vi "修改绑定信息.vi"(9 "修改信息":cluster{"职类":i32, "姓名":string}, 10 "用户名":string, 11 "数据库连接引用":T1) -> (0 "error out":errorcluster)   [LabVIEW 2013, in "数据库操作.lvclass"]
uses:
  <vilib>/addons/database/Connection.llb/Conn ObjectReference.ctl
  <vilib>/addons/database/Connection.llb/Conn Execute.vi
  <vilib>/addons/database/NI_Database_API.lvlib
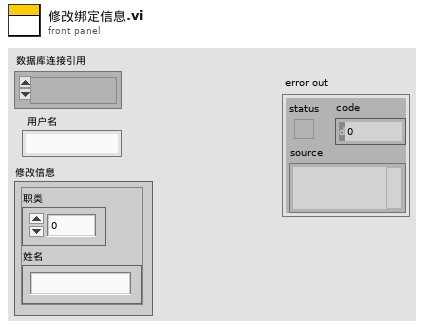
[diagram p1: front panel]
types:
  T1 = typedef "NI_Database_API.lvlib/Conn ObjectReference.ctl" = refnum<k1>
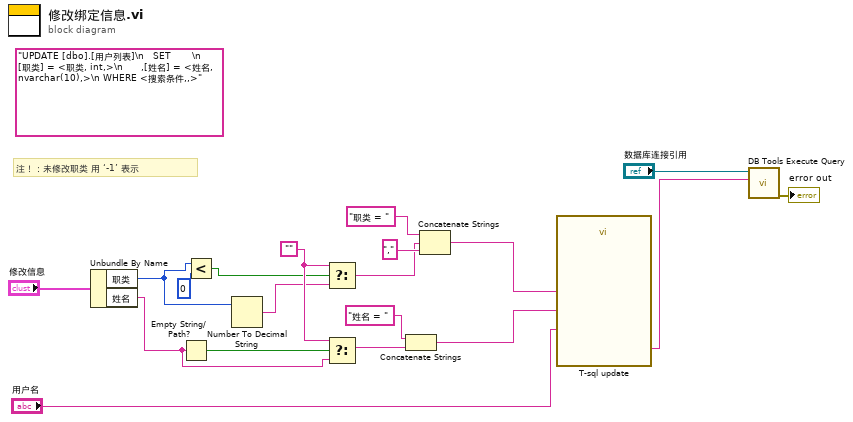
[diagram p0: block diagram]
diagram:
  w17 = ""
  (unwired) "UPDATE [dbo].[用户列表]\n   SET       \n      [职类] = <职类, int,>\n      ,[姓名] = <姓名, nvarchar(10),>\n WHERE <搜索条件,,>"
  # "注！：未修改职类 用 ‘-1’ 表示"
  n1 = Unbundle By Name("修改信息") -> ("职类"=w14:i32, "姓名"=w12:string)
  n2 = Empty String/Path?(string/path=w12) -> (empty?=w15:bool)
  n3 = Less?(x=w14, y=0) -> (x < y?=w16:bool)
  n4 = Number To Decimal String(number=w14) -> (decimal integer string=w13:string)  [unwired: 1 in]
  n5 = Select(t=w17, s=w16, f=w13) -> (s? t:f=w10:string)
  n6 = Select(t=w17, s=w15, f=w12) -> (s? t:f=w9:string)
  n7 = Concatenate Strings("姓名 = " ("字符串"), w9) -> (w5:string)
  n8 = Concatenate Strings("职类 = " ("字符串"), w10, ",") -> (w6:string)
  n9 = call "T-sql update"("职类"=w6, "姓名"=w5, "用户名"="用户名") -> ("Result"=w1:string)  [unwired: 11 in, 1 out]
  n10 = call-poly <vilib>:"DB Tools Execute Query.vi"("SQL query"=w1, "connection reference"="数据库连接引用") -> ("error out"=→"error out":errorcluster)  [unwired: 6 in, 1 out]
